vi "VarifyDataTarget.vi"(8 "error in (no error)":errorcluster, 10 "Destination":string, 11 "GRMActor in":refnum<class "GenericController.lvclass">) -> (0 "error out":errorcluster, 2 "Response?":bool, 3 "GRMActor out":refnum<class "GenericController.lvclass">)   [LabVIEW 2020, in "GenericController.lvlib" / "GenericController.lvclass"]
uses:
  GenericController.lvclass
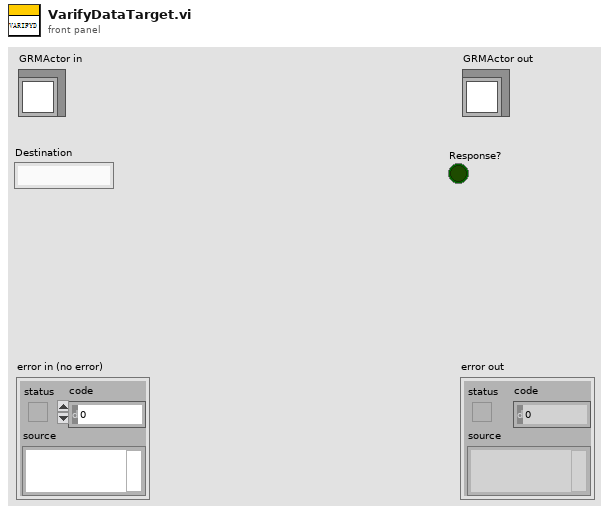
[diagram p1: front panel]
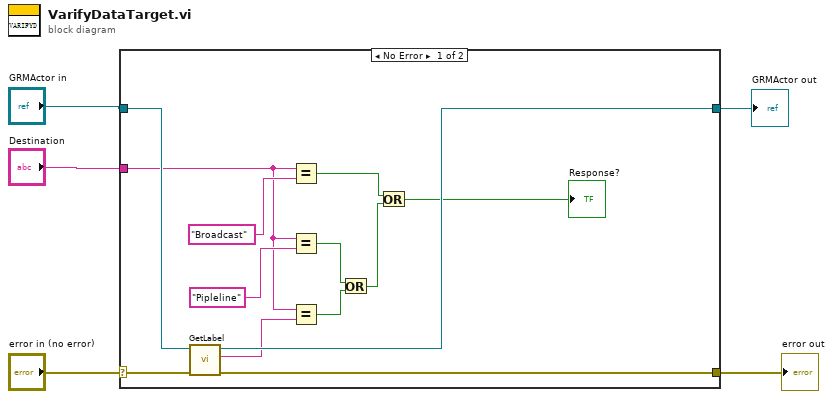
[diagram p0: block diagram]
diagram:
  n1 = case shown="No Error" "error in (no error)" {
    selector: "error in (no error)" -> [w18 w20]
    tunnel: [w17 w20] -> w3
    tunnel: [w15 w19] -> w2
    tunnel: "GRMActor in" -> [w16 w19]
    tunnel: "Destination" -> [w11 _]
    frame No Error {
      n2 = call-dynamic "GetLabel.vi"("error in (no error)"=w18, "GRMActor in"=w16) -> ("error out"=w17:errorcluster, "Label"=w14:string, "GRMActor out"=w15:refnum<class "GenericController.lvclass">)  [unwired: 7 in]
      n3 = Equal?(x=w11, y="Broadcast" ("x")) -> (x = y?=w8:bool)
      n4 = Equal?(x=w11, y="Pipleline") -> (x = y?=w9:bool)
      n5 = Equal?(x=w11, y=w14) -> (x = y?=w10:bool)
      n6 = Or(x=w9, y=w10) -> (x .or. y?=w7:bool)
      n7 = Or(x=w8, y=w7) -> (x .or. y?=→"Response?":bool)
    }
    frame Error {
    }
  }
  "error out" <- w3
  "GRMActor out" <- w2
